vi "Agilent 34401 Read Single Measurement.vi"() -> ()   [LabVIEW 2021]
doc: "This example shows how to configure a measurement and take a single reading."
uses:
  <instrlib>/Agilent 34401/Public/Data/Read (Single Point).vi
  <instrlib>/Agilent 34401/Agilent 34401.lvlib
panel:
  in  "error in":errorcluster
  out "error out":errorcluster
  in  "Function (0: DC Voltage)":u16(ring) items=["DC Voltage", "AC Voltage", "2 - Wire Resistance", "4 - Wire Resistance", "DC Current", "AC Current", "Frequency", "Period", "Continuity", "Diode Checking", "VDC:VDC Ratio", "Temperature", "Capacitance"]
  in  "Manual Range (1.00)":dbl=1.0 format="%_3f"
  in  "Manual Resolution (5.5 Digits)":dbl(ring)=5.5 items=["4.5"=4.5, "5.5"=5.5, "6.5"=6.5]
  in  "Enable Auto Range (T: Enable)":bool=TRUE
  out "Measurement":dbl
  in  "VISA resource name":refnum<visa-resource-name>
  # "(c) 2005-2015 National Instruments.  ALL RIGHTS RESERVED."
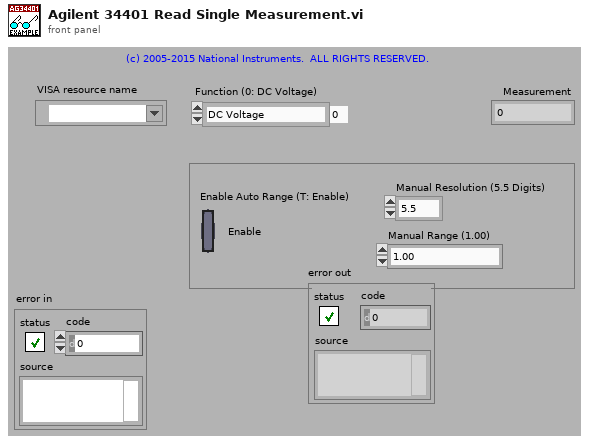
[diagram p1: front panel]
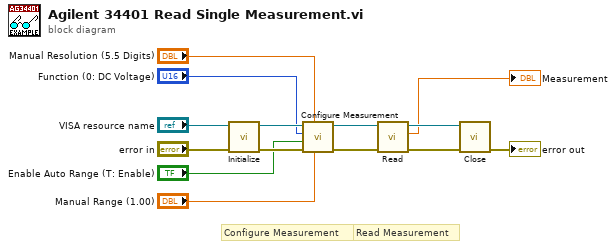
[diagram p0: block diagram]
diagram:
  # "Read Measurement"
  # "Configure Measurement"
  n1 = call <instrlib>:"Initialize.vi"("error in (no error)"="error in", "VISA resource name"="VISA resource name") -> ("error out"=w7:errorcluster, "VISA resource name out"=w8:refnum<visa-resource-name>)  [unwired: 8 in]
  n2 = call <instrlib>:"Configure Measurement.vi"("Manual Range (1.00)"="Manual Range (1.00)", "Manual Resolution (5.5 Digits)"="Manual Resolution (5.5 Digits)", "error in (no error)"=w7, "Enable Auto Range (T: Enable)"="Enable Auto Range (T: Enable)", "Function (0: DC Voltage)"="Function (0: DC Voltage)", "VISA resource name"=w8) -> ("error out"=w9:errorcluster, "VISA resource name out"=w10:refnum<visa-resource-name>)  [unwired: 4 in]
  n3 = call-poly <instrlib>:"Read.vi"("error in (no error)"=w9, "VISA resource name"=w10) -> ("error out"=w13:errorcluster, "Measurement"=→"Measurement":dbl, "VISA resource name out"=w12:refnum<visa-resource-name>)  [unwired: 7 in]
  n4 = call <instrlib>:"Close.vi"("error in (no error)"=w13, "VISA resource name"=w12) -> ("error out"=→"error out":errorcluster)  [unwired: 9 in]
